vi "Configure Trigger (Runt).vi"(6 "Pulse Width (2E-8 S)":dbl=2e-08, 7 "Polarity (0: Positive)":i32(ring) items=["Positive", "Negative", "Either"], 8 "error in (no error)":errorcluster, 9 "Qualifier (0: Greater Than)":i32(ring) items=["Greater Than", "Less Than", "None"], 10 "Trigger Source (0: Channel 1)":i32(ring) items=["Channel 1", "Channel 2", "Channel 3", "Channel 4"], 11 "VISA resource name":refnum<visa-resource-name>) -> (0 "error out":errorcluster, 3 "VISA resource name out":refnum<visa-resource-name>)   [LabVIEW 2015, in "Agilent 2000 3000 X-Series.lvlib"]
doc: "Configures the runt trigger mode.\n\nNote:\nThis VI is not supported by EDUX1052A/G, DSOX1202A/G, DSOX1204A/G models"
uses:
  Agilent 2000 3000 X-Series.lvlib
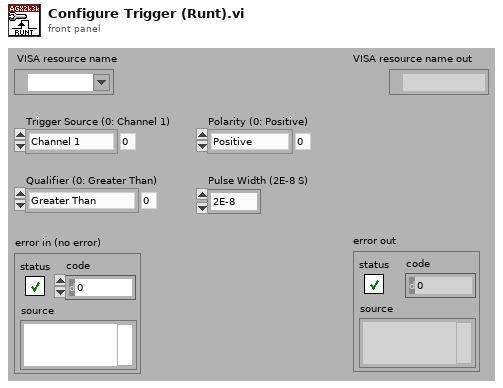
[diagram p1: front panel]
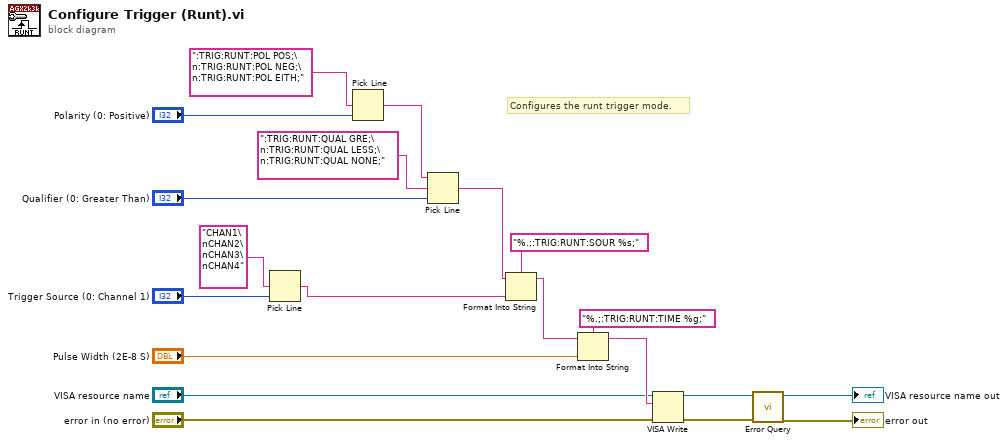
[diagram p0: block diagram]
diagram:
  # "Configures the runt trigger mode."
  n1 = Pick Line(multi-line string="CHAN1\nCHAN2\nCHAN3\nCHAN4", line index="Trigger Source (0: Channel 1)") -> (output string=w1:string)  [unwired: 1 out]
  n2 = Pick Line(multi-line string=":TRIG:RUNT:POL POS;\n:TRIG:RUNT:POL NEG;\n:TRIG:RUNT:POL EITH;", line index="Polarity (0: Positive)") -> (output string=w16:string)  [unwired: 1 out]
  n3 = Pick Line(string ("")=w16, multi-line string=":TRIG:RUNT:QUAL GRE;\n:TRIG:RUNT:QUAL LESS;\n:TRIG:RUNT:QUAL NONE;", line index="Qualifier (0: Greater Than)") -> (output string=w5:string)
  n4 = Format Into String(format string="%.;:TRIG:RUNT:SOUR %s;", initial string=w5, w1) -> (resulting string=w4:string)  [unwired: 1 in, 1 out]
  n5 = Format Into String(format string="%.;:TRIG:RUNT:TIME %g;", initial string=w4, "Pulse Width (2E-8 S)") -> (resulting string=w13:string)  [unwired: 1 in, 1 out]
  n6 = VISA Write(VISA resource name="VISA resource name", write buffer=w13, error in (no error)="error in (no error)") -> (VISA resource name out=w10:refnum<visa-resource-name>, error out=w9:errorcluster)  [unwired: 1 out]
  n7 = call "Error Query.vi"("error in (no error)"=w9, "VISA resource name"=w10) -> ("error out"=→"error out":errorcluster, "VISA resource name out"=→"VISA resource name out":refnum<visa-resource-name>)  [unwired: 8 out]
